vi "set_bearer_auth.vi"(8 "error in":errorcluster, 10 "token":string, 11 "obj in":refnum<class "RequestBuilder.lvclass">) -> (0 "error out":errorcluster, 2 "success":bool, 3 "obj out":refnum<class "RequestBuilder.lvclass">)   [LabVIEW 2020, in "reqwest.lvlib" / "RequestBuilder.lvclass"]
uses:
  RequestBuilder.lvclass
  RequestBuilder.lvclass/RequestBuilder.ctl
  lv_reqwest_64.so
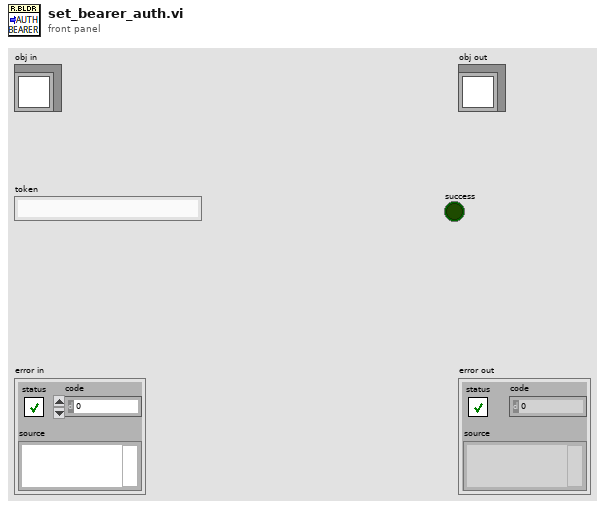
[diagram p1: front panel]
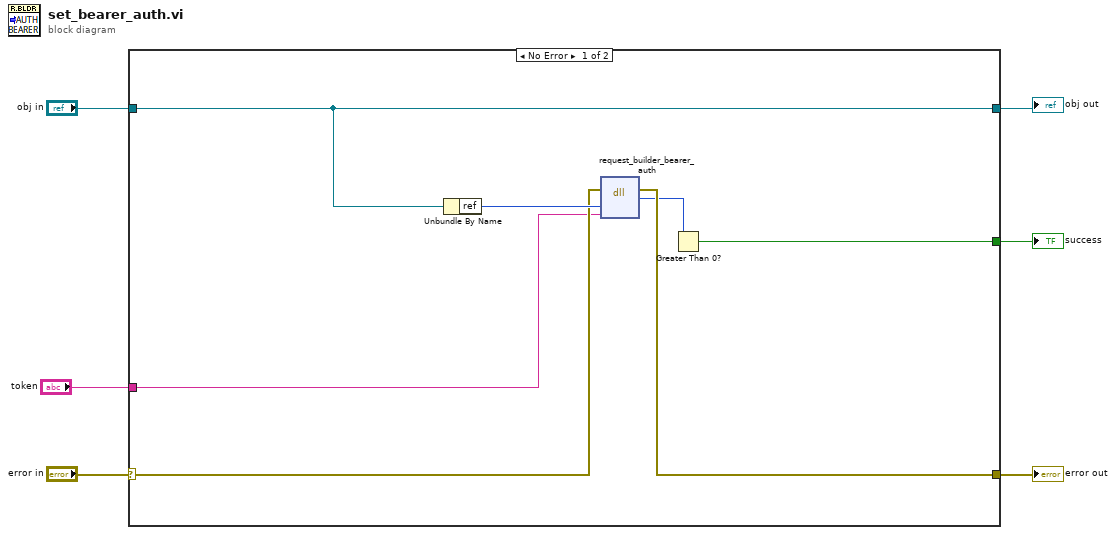
[diagram p0: block diagram]
diagram:
  n1 = case shown="No Error" "error in" {
    selector: "error in" -> [w10 w14]
    tunnel: "obj in" -> [w11 w15]
    tunnel: [w13 w14] -> w3
    tunnel: [w11 w15] -> w4
    tunnel: [w8 _] -> w2
    tunnel: "token" -> [w7 _]
    frame No Error {
      n2 = Unbundle By Name(w11) -> ("ref"=w12:u64)
      n3 = dll-call lib="home/jim-kring/Projects/reqwest-rs-labview/lv_src/lv_reqwest_*.*" fn="request_builder_bearer_auth"(error in=w10, "request_builder_ref"=w12, "token"=w7) -> (error out=w13:errorcluster, "success"=w9:u8)  [unwired: 4 in, 1 out]
      n4 = Greater Than 0?(x=w9) -> (x > 0?=w8:bool)
    }
    frame Error {
    }
  }
  "error out" <- w3
  "obj out" <- w4
  "success" <- w2
